vi "Doublelift to Integerlift.vi"(1 "Double":dbl) -> (0 "Integer":i32)   [LabVIEW 2015]
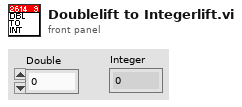
[diagram p1: front panel]
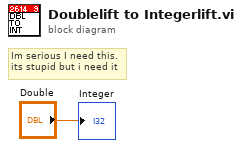
[diagram p0: block diagram]
diagram:
  # "Im serious I need this.\nits stupid but i need it"
  "Integer" <- "Double"
